vi "Command & Ack - Destroy Endpoints.vi"(8 "error in (no error)":errorcluster, 11 "SV B-M (Host) in":refnum<class "SV B-M (Host).lvclass">) -> (0 "error out":errorcluster, 3 "SV B-M (Host) out":refnum<class "SV B-M (Host).lvclass">)   [LabVIEW 2015, in "SV B-M (Host).lvclass"]
doc: "Destroy command & ack network streams."
uses:
  SV B-M (Host).lvclass
  SV B-M (Host).lvclass/SV B-M (Host).ctl
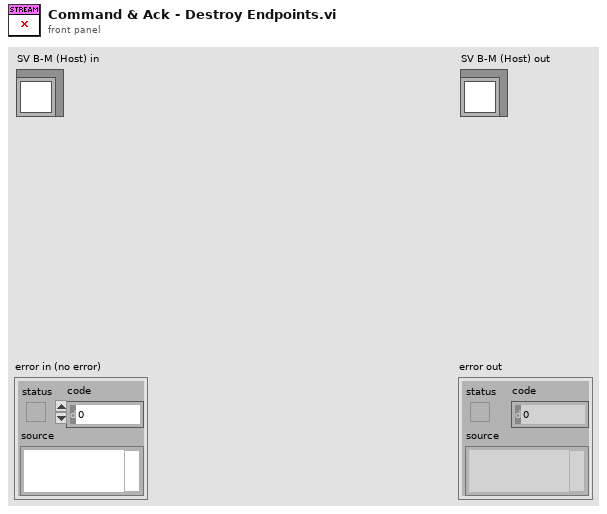
[diagram p1: front panel]
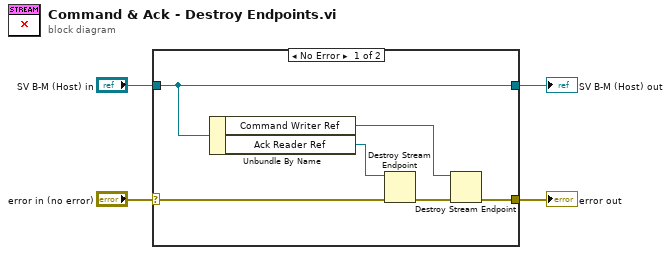
[diagram p0: block diagram]
diagram:
  n1 = case shown="No Error" "error in (no error)" {
    selector: "error in (no error)" -> [w9 w12]
    tunnel: [w5 w12] -> w3
    tunnel: [w10 w11] -> w1
    tunnel: "SV B-M (Host) in" -> [w10 w11]
    frame No Error {
      n2 = Unbundle By Name(w10) -> ("Command Writer Ref"=w7:refnum<k21>, "Ack Reader Ref"=w8:refnum<k21>)
      n3 = Destroy Stream Endpoint(8:w9, 11:w8) -> (0:w6:errorcluster)
      n4 = Destroy Stream Endpoint(8:w6, 11:w7) -> (0:w5:errorcluster)
    }
    frame Error {
    }
  }
  "error out" <- w3
  "SV B-M (Host) out" <- w1
